vi "Read HK Data.vi"(8 "error in (no error)":errorcluster, 11 "Update Housekeeping MSG in":refnum<class "Update Housekeeping MSG.lvclass">) -> (0 "error out":errorcluster, 2 "HK Data":T1(array[cluster]), 3 "Update Housekeeping MSG out":refnum<class "Update Housekeeping MSG.lvclass">)   [LabVIEW 2014, in "eCRDS Library.lvlib" / "Update Housekeeping MSG.lvclass"]
uses:
  Update Housekeeping MSG.lvclass
  Update Housekeeping MSG.lvclass/Update Housekeeping MSG.ctl
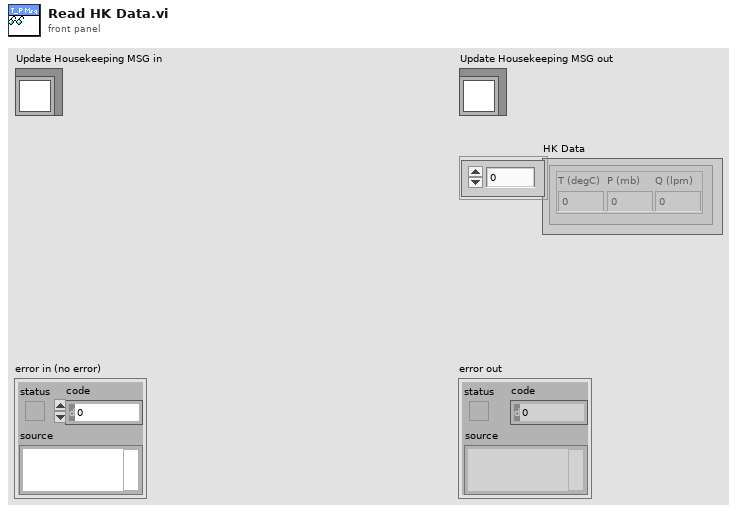
[diagram p1: front panel]
types:
  T1 = cluster{"T (degC)":dbl, "P (mb)":dbl, "Q (lpm)":dbl}[]
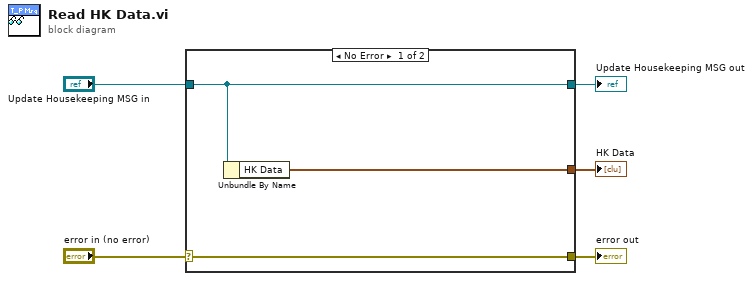
[diagram p0: block diagram]
diagram:
  n1 = case shown="No Error" "error in (no error)" {
    selector: "error in (no error)" -> [w8 w9]
    tunnel: [w8 w9] -> w4
    tunnel: [w7 w10] -> w2
    tunnel: "Update Housekeeping MSG in" -> [w7 w10]
    tunnel: [w6 _] -> w1
    frame No Error {
      n2 = Unbundle By Name(w7) -> ("HK Data"=w6:T1)
    }
    frame Error {
    }
  }
  "error out" <- w4
  "Update Housekeeping MSG out" <- w2
  "HK Data" <- w1
